vi "Merge get section.vi"   [LabVIEW 2020, in "TOML.lvlib"]
uses:
  TOML.lvlib
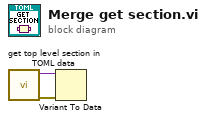
[diagram p0: block diagram]
diagram:
  n1 = call "get top level section in TOML data.vi"() -> ("error out"=w3:errorcluster, "LV Value"=w2:variant, "Section datatype"=w1:variant)  [unwired: 8 in, 1 out]
  n2 = Variant To Data(error in=w3, type=w1, Variant=w2) -> ()  [unwired: 2 out]
